vi "fog.vi"(5 "VISA1":refnum<visa-resource-name>="COM40") -> ()   [LabVIEW 2014]
uses:
  <vilib>/Instr/_visa.llb/VISA Configure Serial Port (Instr).vi
panel:
  in  "stop":bool
  in  "baud rate":u32=9600
  in  "items/line":i32=9
  out "y":dbl
  # "joint angle"
  # "Set Up Communication"
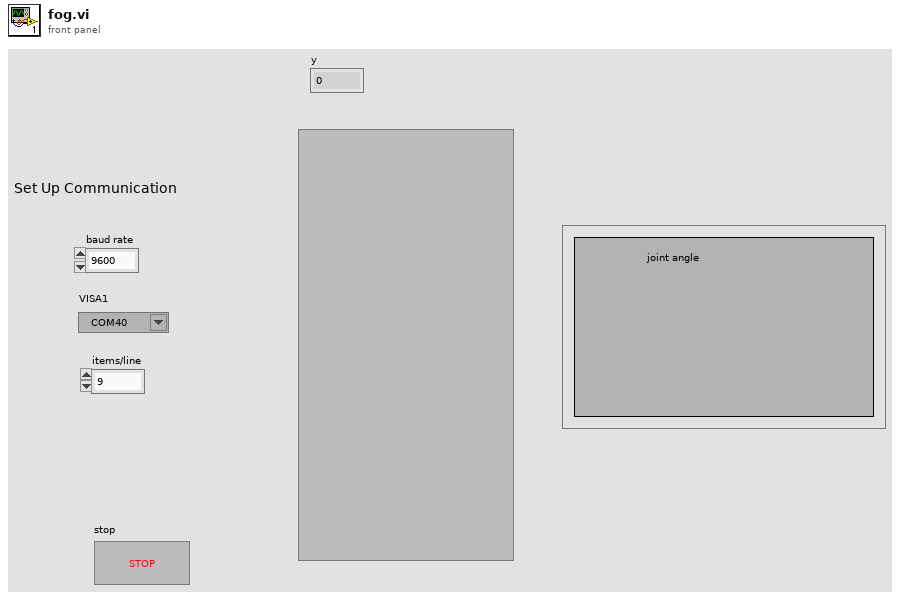
[diagram p1: front panel]
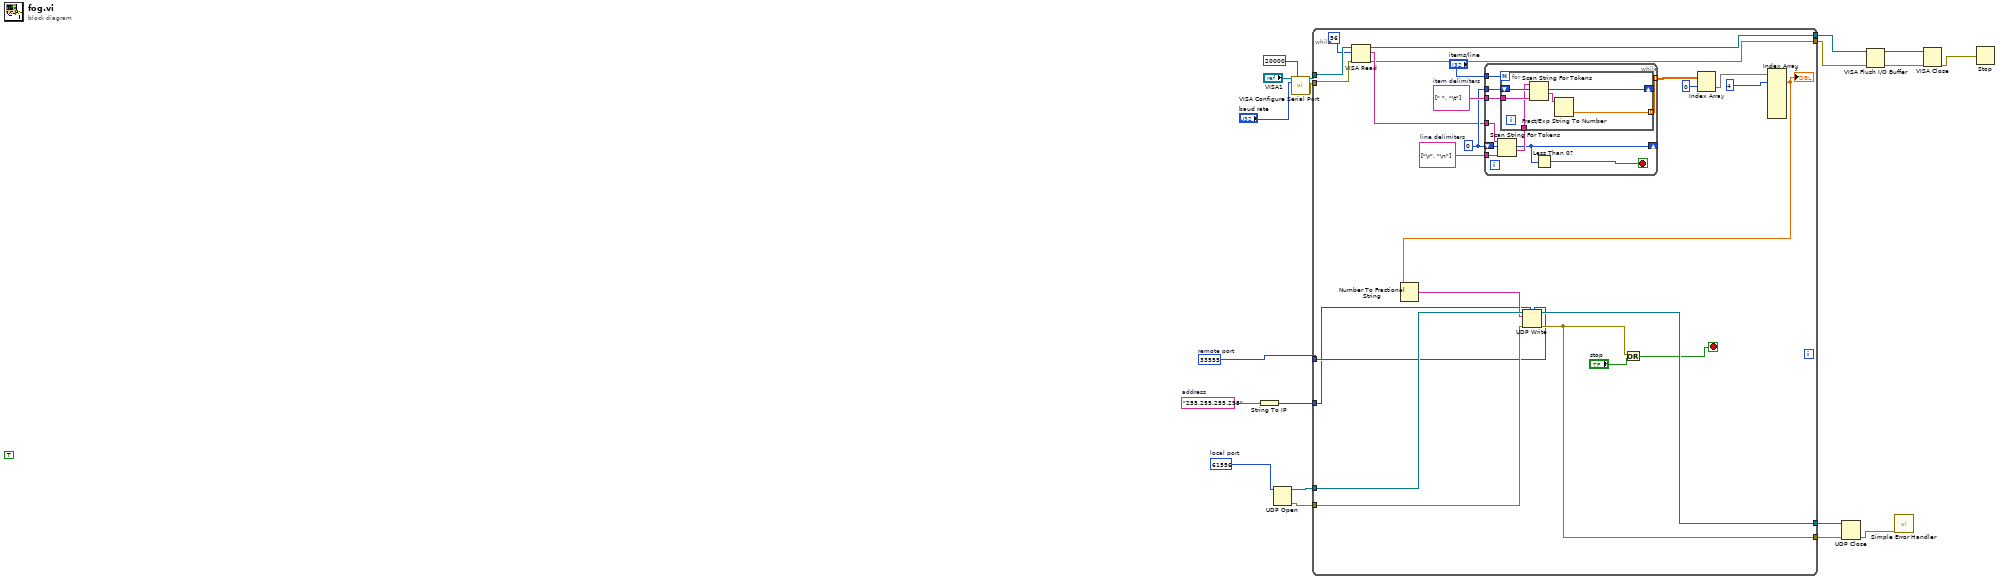
[diagram p0: block diagram]
diagram:
  w4 = u16 33555  # remote port
  w6 = "255.255.255.255"  # address
  w7 = u16 61556  # local port
  (unwired) TRUE ("Visible")
  n1 = String To IP(1:w6) -> (0:w5:u32)
  n2 = UDP Open(11:w7) -> (port=w8:refnum<k16>, 0:w9:errorcluster)  [unwired: 4 in, 1 out]
  n3 = call-poly "VISA Configure Serial Port"("VISA resource name"="VISA1", "timeout (10sec)"=u32 20000, "baud rate (9600)"="baud rate") -> ("VISA resource name out"=w18:refnum<visa-resource-name>, "error out"=w19:errorcluster)  [unwired: 11 in]
  n4 = while {
    tunnel: w18 -> [w43]
    tunnel: [w31] -> w11
    tunnel: w19 -> [w42]
    tunnel: [w30] -> w14
    tunnel: w9 -> [w29]
    tunnel: w8 -> [w28]
    tunnel: w5 -> [w21]
    tunnel: [w27] -> w2
    tunnel: [w26] -> w3
    tunnel: w4 -> [w25]
    stop <- w24 stop-if-true
    w39 = string[] [" ", "\t"]  # item delimiters
    w40 = string[] ["\r", "\n"]  # line delimiters
    w38 = 0 ("offset past token")
    n5 = VISA Read(VISA resource name=w43, byte count=u32 56, error in (no error)=w42) -> (VISA resource name out=w31:refnum<visa-resource-name>, read buffer=w34:string, error out=w30:errorcluster)  [unwired: 1 out]
    n6 = while {
      shift-right: [w49] -> _
      shift-left: w38 -> [w53]
      tunnel: w40 -> [w52]
      tunnel: w39 -> [w51]
      tunnel: w38 -> [w48]
      tunnel: [w47] -> w35 mode=indexing
      tunnel: w34 -> [w46]
      tunnel: "items/line" -> [w45]
      stop <- w44 stop-if-true
      n7 = Scan String For Tokens(6:w52, 8:w53, 9:w46) -> (1:w50:string, 2:w49:i32)  [unwired: 3 in, 2 out]
      n8 = for {
        N: w45 -> [_]
        shift-right: [w58] -> _
        shift-left: w48 -> [w59]
        tunnel: w51 -> [w57]
        tunnel: w50 -> [w56]
        tunnel: [w54] -> w47 mode=indexing
        n9 = Scan String For Tokens(6:w57, 8:w59, 9:w56) -> (1:w55:string, 2:w58:i32)  [unwired: 3 in, 2 out]
        n10 = Fract/Exp String To Number(string=w55) -> (number=w54:dbl)  [unwired: 3 in, 1 out]
      }
      n11 = Less Than 0?(x=w49) -> (x < 0?=w44:bool)
    }
    n12 = Index Array(array=w35, index (row)=0) -> (element=w33:dbl[])  [unwired: 1 in]
    n13 = Index Array(array=w33, index #1=4 ("index")) -> (element #1=w23:dbl)  [unwired: 7 in, 7 out]
    "y" <- w23
    n14 = Number To Fractional String(number=w23) -> (F-format string=w22:string)  [unwired: 3 in]
    n15 = UDP Write(address=w21, port or service name=w25, connection ID=w28, data in=w22, 8:w29) -> (error out=w27:errorcluster, 3:w26:refnum<k16>)  [unwired: 1 in]
    n16 = Or(x=w27, y="stop") -> (x .or. y?=w24:bool)
  }
  n17 = UDP Close(connection ID=w3, 8:w2) -> (error out=w1:errorcluster)  [unwired: 1 out]
  n18 = VISA Flush I/O Buffer(VISA resource name=w11, error in (no error)=w14) -> (VISA resource name out=w13:refnum<visa-resource-name>, error out=w12:errorcluster)  [unwired: 1 in]
  n19 = call <vilib>:"Simple Error Handler.vi"("error in (no error)"=w1) -> ()  [unwired: 4 in, 5 out]
  n20 = VISA Close(VISA resource name=w13, error in (no error)=w12) -> (error out=w10:errorcluster)
  n21 = Stop(stop? (T)=w10) -> ()
